vi "LVCAM Create Nest.vi"(9 "Alias":string, 10 "Nest Actor":refnum<class "LVCAM.lvclass">, 11 "Process in":refnum<class "Process.lvclass">) -> (0 "error out":errorcluster, 3 "Process out":refnum<class "Process.lvclass">)   [LabVIEW 2021, in "Process.lvlib" / "Process.lvclass"]
uses:
  Process.lvclass
  LVCAM/LVCAM/LVCAM/LVCAM.lvclass
  Process.lvclass/Process.ctl
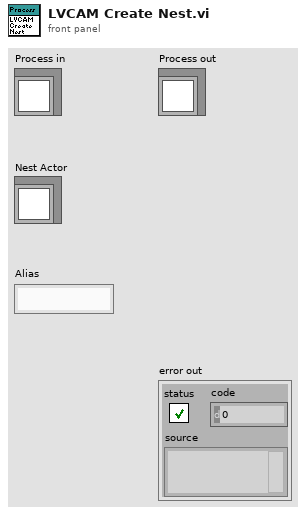
[diagram p1: front panel]
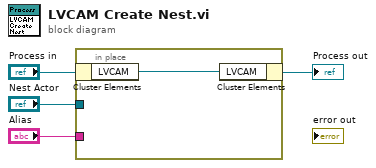
[diagram p0: block diagram]
diagram:
  n1 = in-place {
    in-place-border: "Nest Actor" -> [_]
    in-place-border: "Alias" -> [_]
    n2 = in-place-cluster #1("Process in") -> ("LVCAM"=w5:refnum<class "LVCAM.lvclass">)
    n3 = in-place-cluster #1("LVCAM"=w5) -> (→"Process out":refnum<class "Process.lvclass">)
  }
